vi "Finish.vi"(8 "error in (no error)":errorcluster, 11 "Two Drivers in":refnum<class "Two Drivers.lvclass">) -> (0 "error out":errorcluster, 3 "Two Drivers out":refnum<class "Two Drivers.lvclass">)   [LabVIEW 2019, in "Joysticks.lvlib" / "Two Drivers.lvclass"]
doc: "Use this method to close the references to the joysticks."
uses:
  Two Drivers.lvclass
  Two Drivers.lvclass/Two Drivers.ctl
  <vilib>/Rock Robotics/WPI/Utilities/WPI_GetSetVariantRefNum.vi
  Joysticks.lvclass
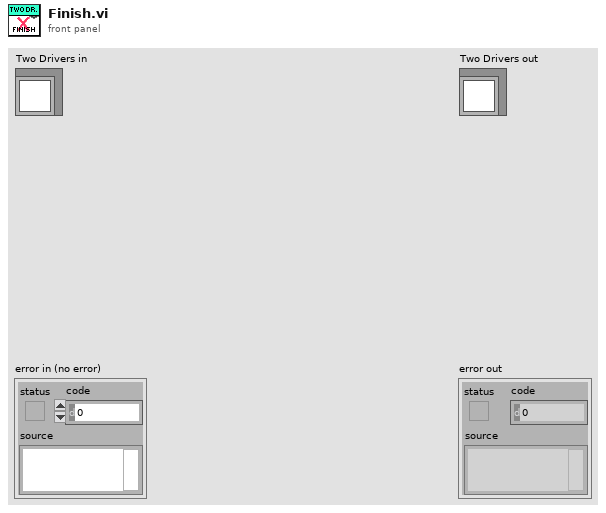
[diagram p1: front panel]
types:
  T1 = typedef "WPI_JoystickDevRef.ctl" = cluster{"Device":T2}
  T2 = typedef "WPI_JoystickDeviceEnum.ctl" = enum16{"USB 0", "USB 1", "USB 2", "USB 3", "USB 4", "USB 5"}
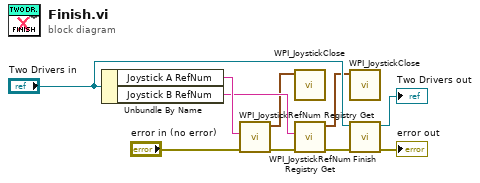
[diagram p0: block diagram]
diagram:
  n1 = Unbundle By Name("Two Drivers in") -> ("Joystick A RefNum"=w4:string, "Joystick B RefNum"=w3:string)
  n2 = call <vilib>:"WPI_JoystickRefNum Registry Get.vi"("error in (no error)"="error in (no error)", "refnum name"=w4) -> ("error out"=w7:errorcluster, "JoystickDevRef"=w2:T1)  [unwired: 8 in]
  n3 = call <vilib>:"WPI_JoystickClose.vi"("JoystickDevRef"=w2) -> ()  [unwired: 11 in]
  n4 = call <vilib>:"WPI_JoystickRefNum Registry Get.vi"("error in (no error)"=w7, "refnum name"=w3) -> ("error out"=w6:errorcluster, "JoystickDevRef"=w1:T1)  [unwired: 8 in]
  n5 = call <vilib>:"WPI_JoystickClose.vi"("JoystickDevRef"=w1) -> ()  [unwired: 11 in]
  n6 = call-parent "Finish.vi"("error in (no error)"=w6, "Joysticks in"="Two Drivers in") -> ("error out"=→"error out":errorcluster, "Joysticks out"=→"Two Drivers out":refnum<class "Two Drivers.lvclass">)  [unwired: 8 in]
